vi "Obtain Message Notifier.vi"(8 "error in (no error)":errorcluster) -> (0 "error out":errorcluster, 3 "Message Notifier":refnum<notifier>)   [LabVIEW 2024, in "DAQ_msgHandler Message Queue.lvlib"]
doc: "Create a queue with the Message Cluster data type."
uses:
  Message Cluster.ctl
  DAQ_msgHandler Message Queue.lvlib
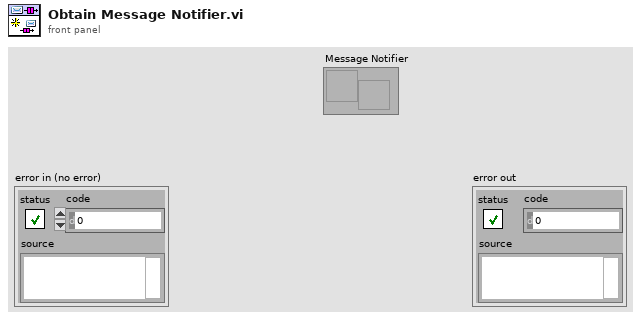
[diagram p1: front panel]
types:
  T1 = typedef "DAQ_msgHandler Message Queue.lvlib/Message Cluster.ctl" = cluster{"Message":string, "Message Data":variant}
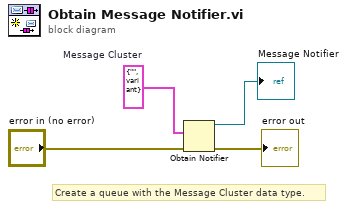
[diagram p0: block diagram]
diagram:
  w4 = T1 {"Message"="", "Message Data"=variant}  # Message Cluster
  # "Create a queue with the Message Cluster data type."
  n1 = Obtain Notifier(notification data type=w4, error in (no error)="error in (no error)") -> (notifier out=→"Message Notifier":refnum<notifier>, error out=→"error out":errorcluster)  [unwired: 2 in, 1 out]
